vi "Preprocess calibration data.vi"(1 "Monotone":bool=TRUE, 2 "Re cal.[]":dbl[](array[numeric]), 3 "X cal.[]":dbl[](array[numeric])) -> (0 "Calibration data":T1)   [LabVIEW 2021]
doc: "Pre-compute the cubic spline interpolating coefficients. Only need to do this once for a given dataset.\nPN 05-NOV-23."
uses:
  Ctls/Calibration data.ctl
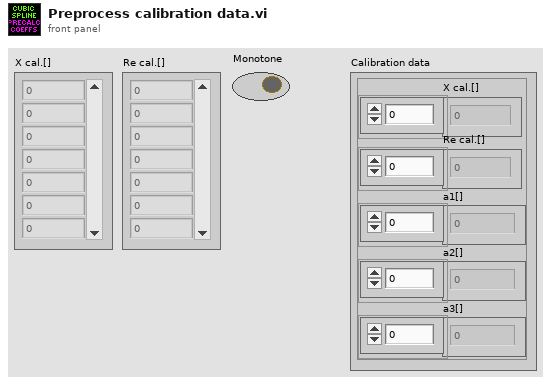
[diagram p1: front panel]
types:
  T1 = typedef "Calibration data.ctl" = cluster{"X cal.[]":dbl[], "Re cal.[]":dbl[], "a1[]":dbl[], "a2[]":dbl[], "a3[]":dbl[]}
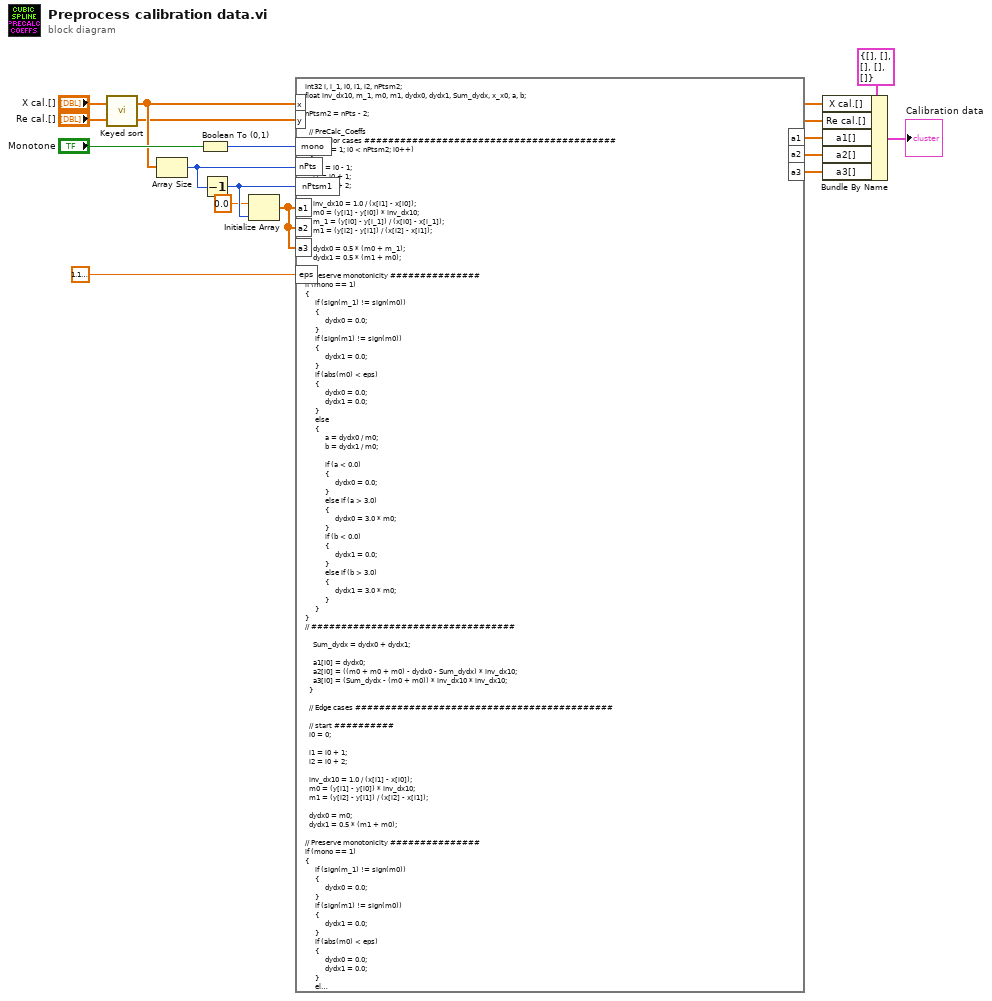
[diagram p0: block diagram]
diagram:
  n1 = call "Keyed sort.vi"("Re cal.[]"="Re cal.[]", "X cal.[]"="X cal.[]") -> ("Re cal. keyed sorted[]"=w1:dbl[], "X cal. sorted[]"=w2:dbl[])
  n2 = Array Size(array=w2) -> (size(s)=w16:i32)
  n3 = Boolean To (0,1)(Boolean="Monotone") -> (0, 1=w14:i16)
  n4 = Decrement(x=w16) -> (x-1=w12:i32)
  n5 = Initialize Array(0.0 ("element"), w12) -> (w10:dbl[])
  n6 = formula code="int32 i, i_1, i0, i1, i2, nPtsm2;\nfloat inv_dx10, m_1, m0, m1, dydx0, dydx1, Sum_dydx, x_x0, a, b;\n\nnPtsm2 = nPts - 2;\n\n  // PreCalc_Coeffs\n  // Interior cases ##########################################\n  for (i0 = 1; i0 < nPtsm2; i0++)\n  {\n    i_1 = i0 - 1;\n    i1 = i0 + 1;\n    i2 = i0 + 2;\n\n    inv_dx10 = 1.0 / (x[i1] - x[i0]);\n    m0 = (y[i1] - y[i0]) * inv_dx10;\n    m_1 = (y[i0] - y[i_1]) / (x[i0] - x[i_1]);\n    m1 = (y[i2] - y[i1]) / (x[i2] - x[i1]);\n\n    dydx0 = 0.5 * (m0 + m_1);\n    dydx1 = 0.5 * (m1 + m0);\n\n// Preserve monotonicity ###############\nif (mono == 1)\n{\n     if (sign(m_1) != sign(m0))\n     {\n          dydx0 = 0.0;\n     }\n     if (sign(m1) != sign(m0))\n     {\n          dydx1 = 0.0;\n     }\n     if (abs(m0) < eps)\n     {\n          dydx0 = 0.0;\n          dydx1 = 0.0;\n     }\n     else\n     {\n          a = dydx0 / m0;\n          b = dydx1 / m0;    \n            \n          if (a < 0.0)\n          {\n               dydx0 = 0.0;\n          }\n          else if (a > 3.0)\n          {\n               dydx0 = 3.0 * m0;\n          }\n          if (b < 0.0)\n          {\n               dydx1 = 0.0;\n          }   \n          else if (b > 3.0)\n          {\n               dydx1 = 3.0 * m0;\n          }\n     }\n}\n// ##################################\n\n    Sum_dydx = dydx0 + dydx1;\n\n    a1[i0] = dydx0;\n    a2[i0] = ((m0 + m0 + m0) - dydx0 - Sum_dydx) * inv_dx10;\n    a3[i0] = (Sum_dydx - (m0 + m0)) * inv_dx10 * inv_dx10;\n  }\n\n  // Edge cases ###########################################\n\n  // start ##########\n  i0 = 0;\n\n  i1 = i0 + 1;\n  i2 = i0 + 2;\n\n  inv_dx10 = 1.0 / (x[i1] - x[i0]);\n  m0 = (y[i1] - y[i0]) * inv_dx10;\n  m1 = (y[i2] - y[i1]) / (x[i2] - x[i1]);\n\n  dydx0 = m0;\n  dydx1 = 0.5 * (m1 + m0);\n\n// Preserve monotonicity ###############\nif (mono == 1)\n{\n     if (sign(m_1) != sign(m0))\n     {\n          dydx0 = 0.0;\n     }\n     if (sign(m1) != sign(m0))\n     {\n          dydx1 = 0.0;\n     }\n     if (abs(m0) < eps)\n     {\n          dydx0 = 0.0;\n          dydx1 = 0.0;\n     }\n     else\n     {\n          a = dydx0 / m0;\n          b = dydx1 / m0;    \n            \n          if (a < 0.0)\n          {\n               dydx0 = 0.0;\n          }\n          else if (a > 3.0)\n          {\n               dydx0 = 3.0 * m0;\n          }\n          if (b < 0.0)\n          {\n               dydx1 = 0.0;\n          }   \n          else if (b > 3.0)\n          {\n               dydx1 = 3.0 * m0;\n          }\n     }\n}\n// ##################################\n\n  Sum_dydx = dydx0 + dydx1;\n\n  a1[i0] = dydx0;\n  a2[i0] = ((m0 + m0 + m0) - dydx0 - Sum_dydx) * inv_dx10;\n  a3[i0] = (Sum_dydx - (m0 + m0)) * inv_dx10 * inv_dx10;\n\n  // end ##########\n  i0 = nPtsm2;\n\n  i_1 = i0 - 1;\n  i1 = i0 + 1;\n\n  inv_dx10 = 1.0 / (x[i1] - x[i0]);\n  m0 = (y[i1] - y[i0]) * inv_dx10;\n  m_1 = (y[i0] - y[i_1]) / (x[i0] - x[i_1]);\n\n  dydx0 = 0.5 * (m0 + m_1);\n  dydx1 = m0;\n\n// Preserve monotonicity ###############\nif (mono == 1)\n{\n     if (sign(m_1) != sign(m0))\n     {\n          dydx0 = 0.0;\n     }\n     if (sign(m1) != sign(m0))\n     {\n          dydx1 = 0.0;\n     }\n     if (abs(m0) < eps)\n     {\n          dydx0 = 0.0;\n          dydx1 = 0.0;\n     }\n     else\n     {\n          a = dydx0 / m0;\n          b = dydx1 / m0;    \n            \n          if (a < 0.0)\n          {\n               dydx0 = 0.0;\n          }\n          else if (a > 3.0)\n          {\n               dydx0 = 3.0 * m0;\n          }\n          if (b < 0.0)\n          {\n               dydx1 = 0.0;\n          }   \n          else if (b > 3.0)\n          {\n               dydx1 = 3.0 * m0;\n          }\n     }\n}\n// ##################################\n\n  Sum_dydx = dydx0 + dydx1;\n\n  a1[i0] = dydx0;\n  a2[i0] = ((m0 + m0 + m0) - dydx0 - Sum_dydx) * inv_dx10;\n  a3[i0] = (Sum_dydx - (m0 + m0)) * inv_dx10 * inv_dx10;\n\n  // ###################################################"("x"=w2, "nPts"=w16, "y"=w1, "nPtsm1"=w12, "mono"=w14, "eps"=sgl 1.1920929e-07, "a1"=w10, "a2"=w10, "a3"=w10) -> ("a1"=w7:dbl[], "a2"=w6:dbl[], "a3"=w5:dbl[])
  n7 = Bundle By Name(cluster=T1 {"X cal.[]"=[], "Re cal.[]"=[], "a1[]"=[], "a2[]"=[], "a3[]"=[]} ("Spline coefficients"), "X cal.[]"=w2, "Re cal.[]"=w1, "a1[]"=w7, "a2[]"=w6, "a3[]"=w5) -> (→"Calibration data":T1)
